vi "ReadExternalPosition.vi"() -> ()   [LabVIEW 2011, in "UnderAutomation.Yaskawa.lvlib"]
uses:
  UnderAutomation.Yaskawa.lvlib
  C:/Users/fg/Documents/Yaskawa.vi/LabVIEW_2024/UnderAutomation.Yaskawa/lib/UnderAutomation.Yaskawa.dll
  LabVIEW_2024/UnderAutomation.Yaskawa/lib/UnderAutomation.Yaskawa.dll
panel:
  out "Axes":i32[][](array[numeric])
  in  "count":i32
  in  "firstIndex":i32
  out "error out":errorcluster
  in  "error in (no error)":errorcluster
  in  "HighSpeedEServer":refnum<k24>
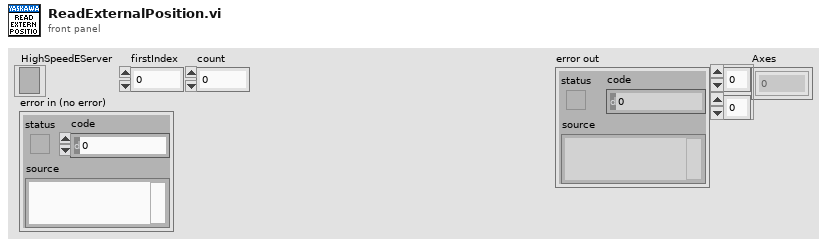
[diagram p1: front panel]
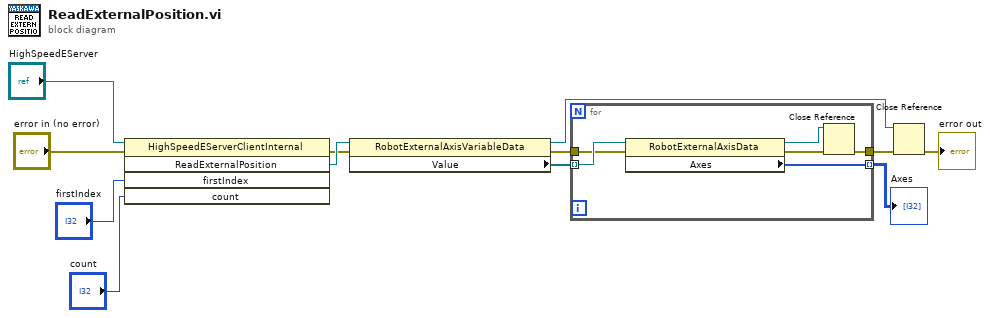
[diagram p0: block diagram]
diagram:
  n1 = invoke class="HighSpeedEServerClientInternal" method="ReadExternalPosition"(reference="HighSpeedEServer", error in="error in (no error)", "firstIndex"="firstIndex", "count"="count") -> (error out=w6:errorcluster, "ReadExternalPosition"=w8:refnum<k24>)  [unwired: 1 in, 3 out]
  n2 = property class="RobotExternalAxisVariableData"(reference=w8, error in=w6) -> (reference out=w7:refnum<k24>, error out=w2:errorcluster, "Value"=w4:refnum<k24>[])
  n3 = for {
    tunnel: w4 -> [w18] mode=indexing
    tunnel: [w17] -> w3 mode=indexing
    tunnel: w2 -> [w14]
    tunnel: [w13] -> w1
    n4 = property class="RobotExternalAxisData"(reference=w18, error in=w14) -> (reference out=w16:refnum<k24>, error out=w15:errorcluster, "Axes"=w17:i32[])
    n5 = Close Reference(reference=w16, error in (no error)=w15) -> (error out=w13:errorcluster)
  }
  "Axes" <- w3
  n6 = Close Reference(reference=w7, error in (no error)=w1) -> (error out=→"error out":errorcluster)
